vi "Error_Helper_OverwriteCluster.vi"(6 "Additional Info":string, 8 "Error In":errorcluster, 11 "Code":i32) -> (0 "Error Out":errorcluster)   [LabVIEW 2020, in "hse-misc.lvlib"]
doc: "If <b>Error In</b> is true, overwrites the error cluster information with <b>Code</b> and <b>Additional Info</b>.\n\n____\nHAMPEL SOFTWARE ENGINEERING v3.8.0 (2023-12-18 14:41)"
uses:
  hse-misc.lvlib
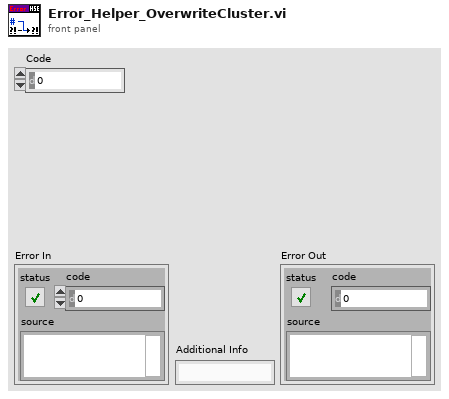
[diagram p1: front panel]
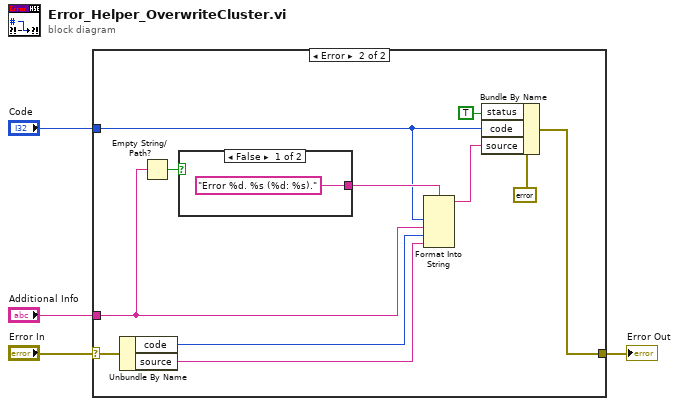
[diagram p0: block diagram]
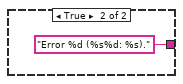
[diagram p3: hidden frame]
diagram:
  n1 = case shown="Error" "Error In" {
    selector: "Error In" -> [w5 w11]
    tunnel: [w5 w16] -> w4
    tunnel: "Code" -> [_ w6]
    tunnel: "Additional Info" -> [_ w10]
    frame No Error {
    }
    frame Error {
      n2 = Unbundle By Name(w11) -> ("code"=w9:i32, "source"=w7:string)
      n3 = Empty String/Path?(string/path=w10) -> (empty?=w13:bool)
      n4 = case shown="False" w13 {
        tunnel: ["Error %d. %s (%d: %s)." ("format string") "Error %d (%s%d: %s)." ("format string")] -> w8
        frame False {
        }
        frame True {
        }
      }
      n5 = Format Into String(format string=w8, w6, w10, w9, w7) -> (resulting string=w12:string)  [unwired: 2 in, 1 out]
      n6 = Bundle By Name(cluster=errorcluster {"status"=TRUE, "code"=0, "source"=""} ("error IO"), "status"=TRUE, "code"=w6, "source"=w12) -> (w16:errorcluster)
    }
  }
  "Error Out" <- w4
